vi "THzTimeScan_830_PSD_TA.vi"(0 "input":T1={"Step Number"=0, "Step"=0.0, "Start Position"=0.0, "Time-out"=0, "Lockin Address"="", "Short term \nAverage#"=0, 0, "ESP300 Axis"=0, "Value"="", "Delay"=0.0, "Delay2"=0.0, "savepath"=path "", "Power meter"={"ConexPSD Reference"=refnum, "error out"={"status"=FALSE, "code"=0, "source"=""}, "Component ID"=1}}) -> (1 "loop stop":bool, 2 "x-axis":sgl[](array[numeric]), 3 "y-axis":dbl[](array[numeric]), 4 "ext. out":cluster{dbl[], dbl[], dbl[], dbl[], string[]})   [LabVIEW 2010]
uses:
  C:/Users/NBTP/Desktop/Tai Anh/5. Tools Project/LabVIEW/노트북LabVIEW/THz Time/THz Time(SR830_VC_CONEXAGP_nPt_Shot202_2Pt__LGS/Dll/Newport.CONEXPSD.CommandInterface.DLL
  노트북LabVIEW/THz Time/THz Time(SR830_VC_CONEXAGP_nPt_Shot202_2Pt__LGS/Dll/Newport.CONEXPSD.CommandInterface.DLL
  <vilib>/Utility/file.llb/Write To Spreadsheet File (string).vi
panel:
  out "Total info.":cluster{dbl, dbl, dbl}(graph)
  in  "y offset":dbl
  in  "x offset":dbl
  out "PD pow.":dbl
  out "Y pos.":dbl
  out "X pos.":dbl
  in  "pow. offset":dbl
  out "Pow.":dbl
  out "Array":dbl[](array[numeric])
  out "String":string
  out "Read position":bool
  out "Ask position":bool
  out "Move delay":bool
  out "Read830":bool
  out "Command":string
  out "THz Signal Graph":dbl(graph)
  in  "loop stop":bool
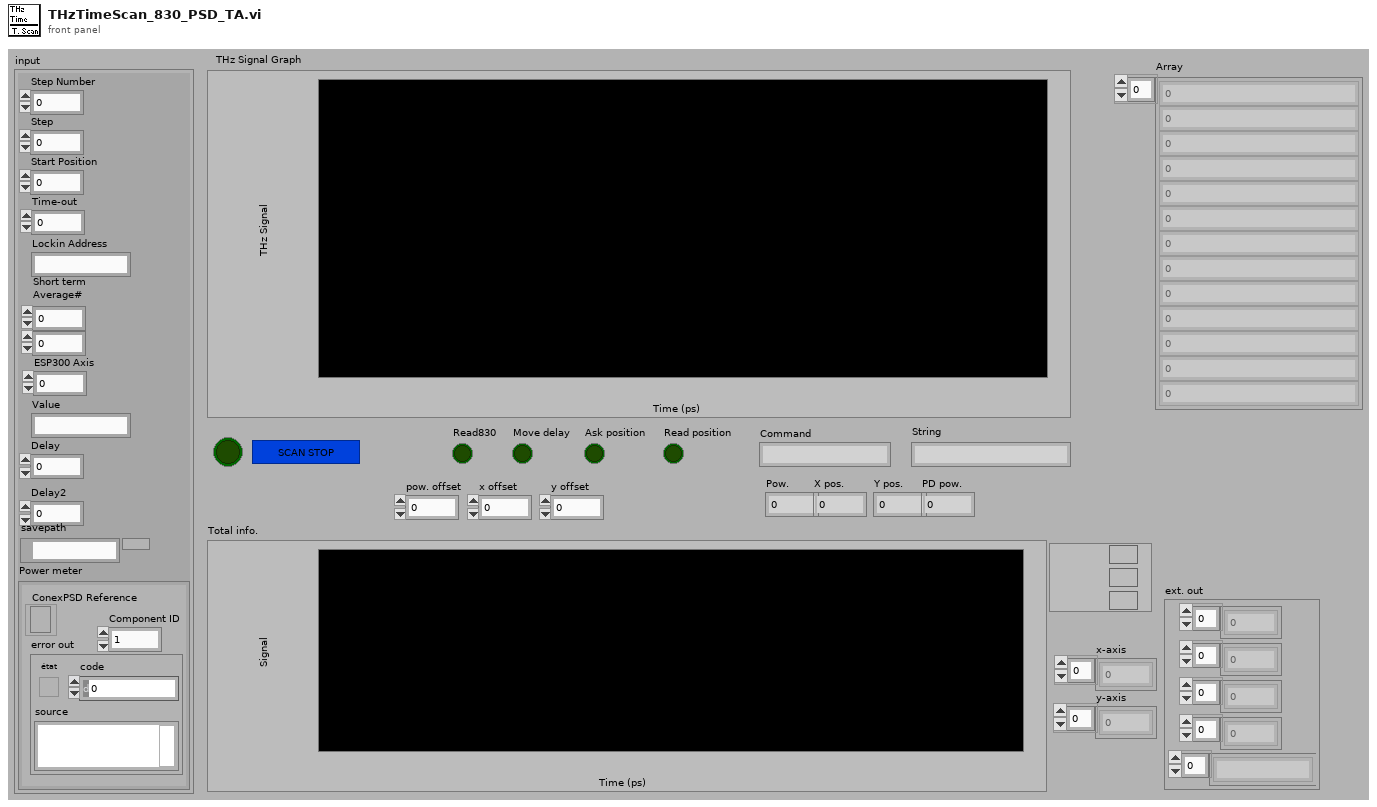
[diagram p1: front panel]
types:
  T1 = cluster{"Step Number":i32, "Step":sgl, "Start Position":sgl, "Time-out":i32, "Lockin Address":string, "Short term \nAverage#":i8, i32, "ESP300 Axis":i8, "Value":string, "Delay":dbl, "Delay2":dbl, "savepath":path, "Power meter":cluster{"ConexPSD Reference":refnum<k24>, "error out":errorcluster, "Component ID":i32}}
  T2 = cluster{"ConexPSD Reference":refnum<k24>, "error out":errorcluster, "Component ID":i32}
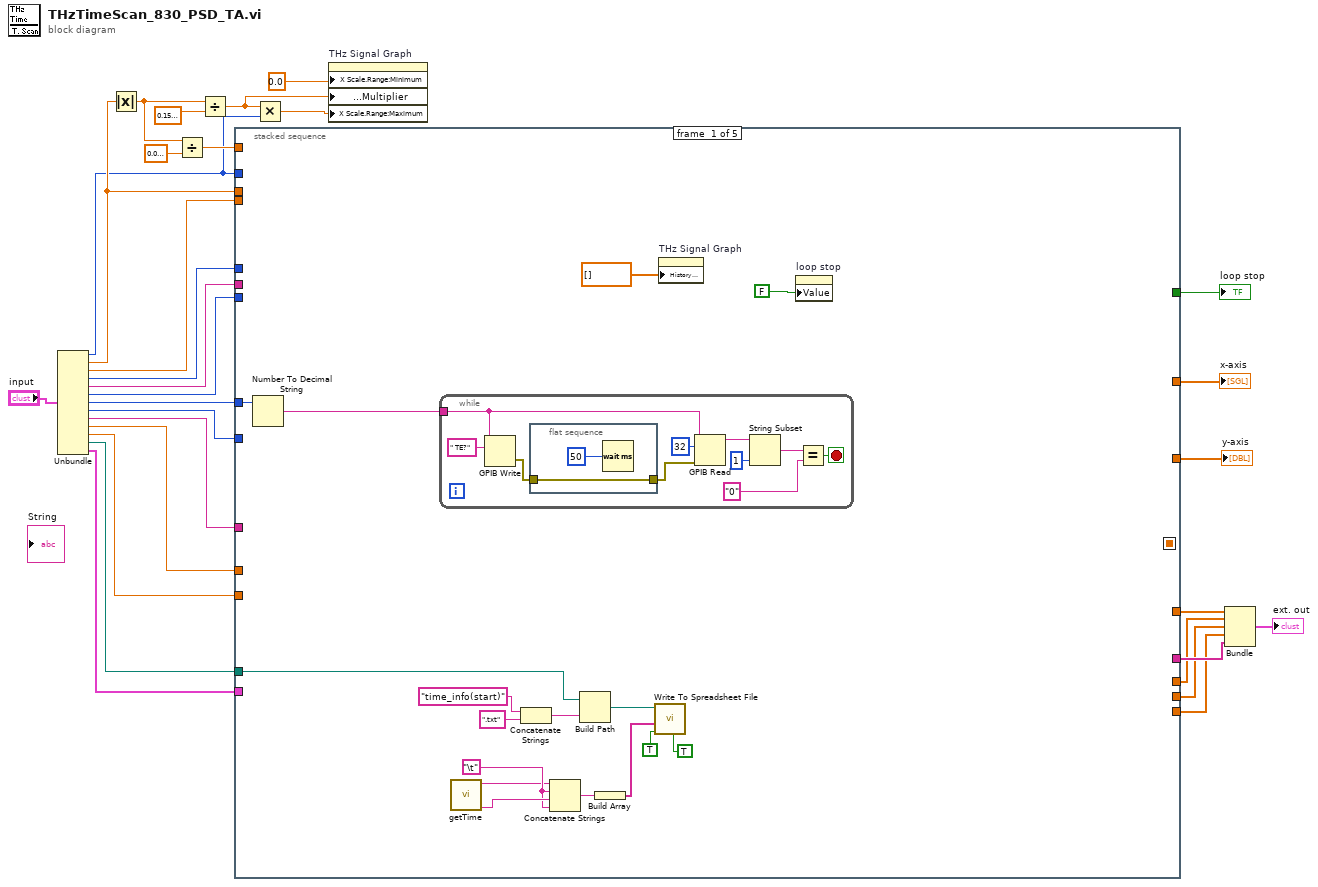
[diagram p0: block diagram]
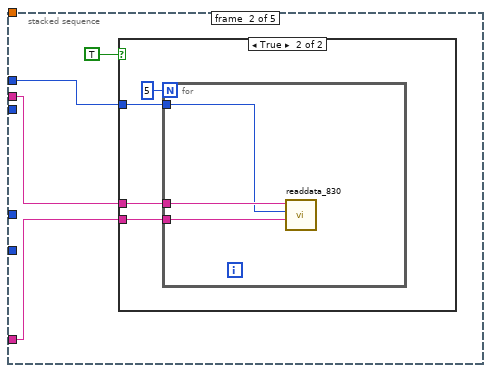
[diagram p2: hidden frame]
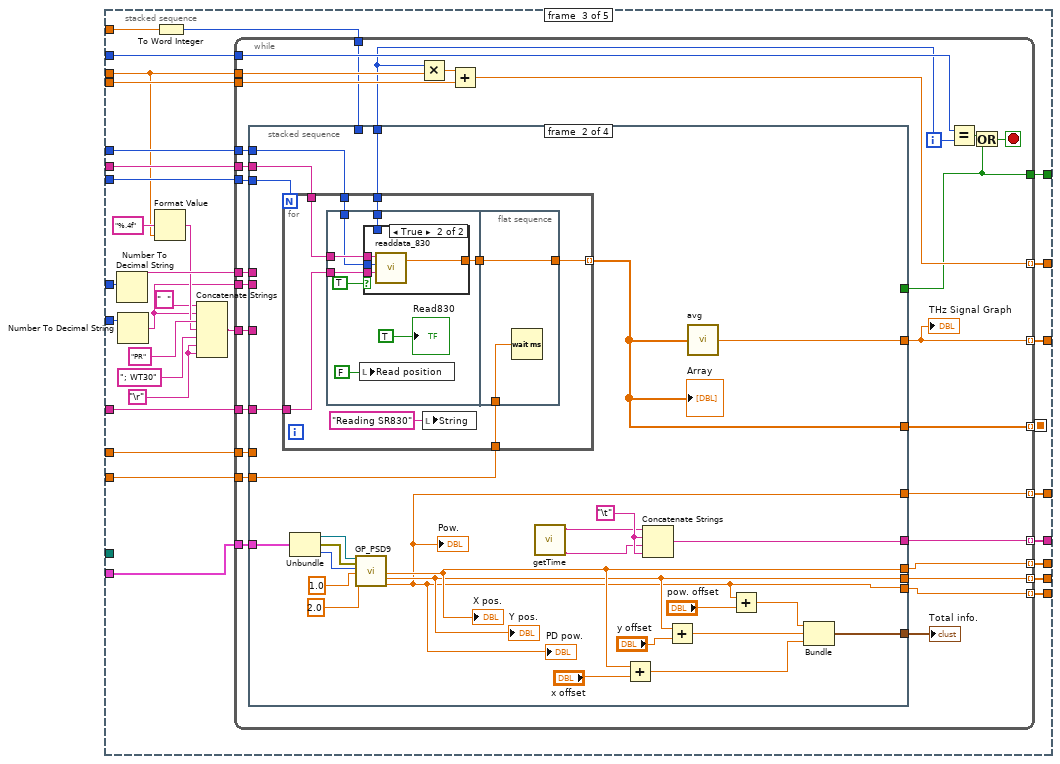
[diagram p4: hidden frame]
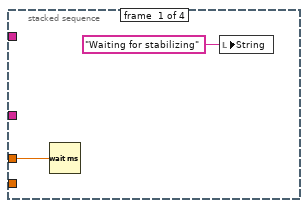
[diagram p5: hidden frame]
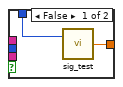
[diagram p6: hidden frame]
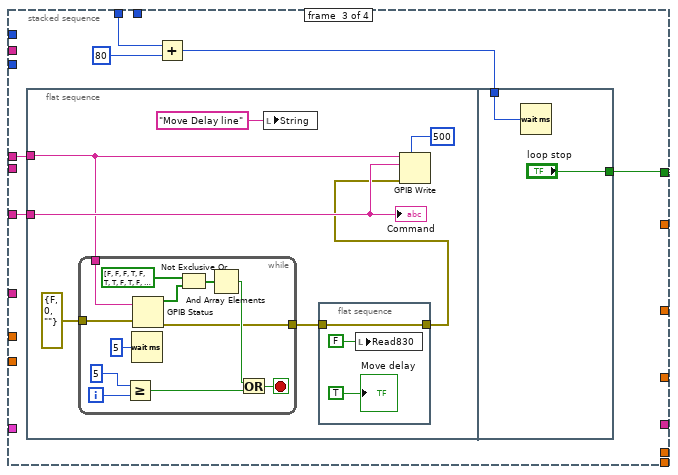
[diagram p7: hidden frame]
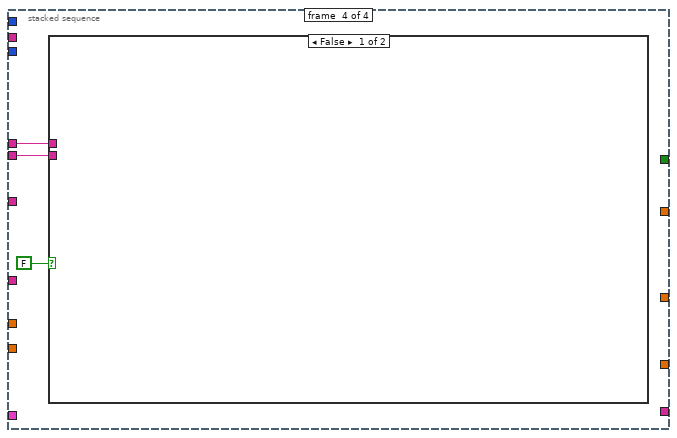
[diagram p8: hidden frame]
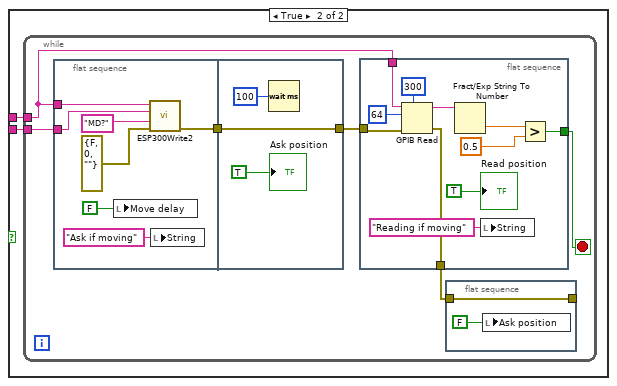
[diagram p9: hidden frame]
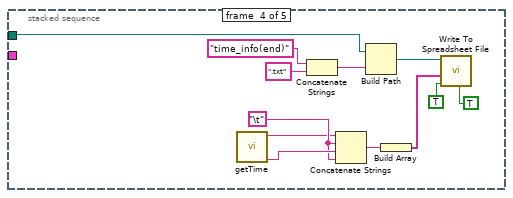
[diagram p10: hidden frame]
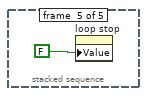
[diagram p11: hidden frame]
diagram:
  n1 = Unbundle("input") -> ("Step Number"=w15:i32, "Step"=w22:sgl, "Start Position"=w21:sgl, "Time-out"=w20:i32, "Lockin Address"=w19:string, "Short term \nAverage#"=w11:i8, w18:i32, "ESP300 Axis"=w17:i8, "Value"=w16:string, "Delay"=w10:dbl, "Delay2"=w9:dbl, "savepath"=w8:path, "Power meter"=w7:T2)
  n2 = Absolute Value(x=w22) -> (abs(x)=w26:sgl)
  n3 = Divide(x=w26, y=sgl 0.004) -> (x/y=w24:sgl)
  n4 = Divide(x=w26, y=sgl 0.15) -> (x/y=w13:sgl)
  n5 = stacked-sequence {
    seq-local: [_ _ w77 _ _] -> [_ _ _ _ _]
    tunnel: w21 -> [_ _ w101 _ _]
    tunnel: w20 -> [_ w62 w100 _ _]
    tunnel: w19 -> [_ w61 w99 _ _]
    tunnel: w11 -> [_ _ w98 _ _]
    tunnel: w18 -> [w44 _ w93 _ _]
    tunnel: w17 -> [_ _ w91 _ _]
    tunnel: w16 -> [_ w60 w83 _ _]
    tunnel: [_ _ w97 _ _] -> w30
    tunnel: [_ _ w96 _ _] -> w29
    tunnel: [_ _ w95 _ _] -> w28
    tunnel: w22 -> [_ _ w89 _ _]
    tunnel: w15 -> [_ _ w94 _ _]
    tunnel: w24 -> [_ _ w88 _ _]
    tunnel: w10 -> [_ _ w79 _ _]
    tunnel: w9 -> [_ _ w78 _ _]
    tunnel: w8 -> [w31 _ _ w248 _]
    tunnel: w7 -> [_ _ w75 _ _]
    tunnel: [_ _ w74 _ _] -> w6
    tunnel: [_ _ w73 _ _] -> w5
    tunnel: [_ _ w72 _ _] -> w4
    tunnel: [_ _ w71 _ _] -> w3
    tunnel: [_ _ w70 _ _] -> w2
    frame #0 {
      w34 = "\t"
      n6 = Number To Decimal String(number=w44) -> (decimal integer string=w43:string)  [unwired: 1 in]
      n7 = while {
        tunnel: w43 -> [w49]
        stop <- w54 stop-if-true
        n8 = GPIB Write(0:w49, 1:" TE?" ("data")) -> (6:w48:errorcluster)  [unwired: 3 in, 1 out]
        n9 = flat-sequence {
          tunnel: w48 -> [w58]
          tunnel: [w58] -> w47
          frame #0 {
            n10 = Wait (ms)(milliseconds to wait=u32 50) -> ()  [unwired: 1 out]
          }
        }
        n11 = GPIB Read(0:w49, 1:32 ("byte count"), 3:w47) -> (5:w53:string)  [unwired: 2 in, 2 out]
        n12 = String Subset(string=w53, length (rest)=1 ("offset (0)")) -> (substring=w51:string)  [unwired: 1 in]
        n13 = Equal?(x=w51, y="0") -> (x = y?=w54:bool)
      }
      n14 = call "getTime.vi"() -> ("시간"=w35:string, "날짜"=w33:string)  [unwired: 10 in]
      n15 = Concatenate Strings("time_info(start)" ("string"), ".txt" ("string")) -> (w41:string)
      n16 = Concatenate Strings(w33, w34, w35, w34) -> (w32:string)
      n17 = Build Path(base path=w31, name or relative path=w41) -> (appended path=w38:path)
      n18 = Build Array(w32) -> (w37:string[])
      n19 = call-poly <vilib>:"Write To Spreadsheet File.vi"("transpose? (no:F)"=TRUE ("transpose?\n(no:F)"), "append to file? (new file:F)"=TRUE ("transpose?\n(no:F)"), "1D data"=w37, "file path (dialog if empty)"=w38) -> ()  [unwired: 4 in, 1 out]
      n20 = property on="THz Signal Graph" class="WFChart (strict)"("History Data"=dbl[] []) -> ()  [unwired: 2 in, 2 out]
      n21 = property on="loop stop" class="Bool (strict)"("Value"=FALSE) -> ()  [unwired: 2 in, 2 out]
    }
    frame #1 {
      n22 = case shown="True" TRUE {
        tunnel: w62 -> [_ w65]
        tunnel: w61 -> [_ w64]
        tunnel: w60 -> [_ w63]
        frame False {
        }
        frame True {
          n23 = for {
            N: 5 -> [_]
            tunnel: w64 -> [w69]
            tunnel: w63 -> [w68]
            tunnel: w65 -> [w67]
            n24 = call "readdata_830.vi"("Command"=w68, "timeout"=w67, "Lockin Address"=w69) -> ()  [unwired: 1 in, 2 out]
          }
        }
      }
    }
    frame #2 {
      w82 = "\r"
      n25 = Number To Decimal String(number=w93) -> (decimal integer string=w92:string)  [unwired: 1 in]
      n26 = Number To Decimal String(number=w91) -> (decimal integer string=w80:string)  [unwired: 1 in]
      n27 = Format Value(format string="%.4f", value (0)=w89) -> (output string=w85:string)  [unwired: 1 in]
      n28 = To Word Integer(number=w88) -> (16bit integer=w87:i16)
      n29 = Concatenate Strings("  " ("string"), w80, "PR" ("Substring"), w85, "; WT30" ("string"), w82, w82) -> (w76:string)
      n30 = while {
        tunnel: [w114] -> w97
        tunnel: [w120] -> w95 mode=indexing
        tunnel: [w126] -> w96 mode=indexing
        tunnel: w94 -> [w125]
        tunnel: w89 -> [w124]
        tunnel: w101 -> [w123]
        tunnel: w100 -> [w115]
        tunnel: w99 -> [w122]
        tunnel: w98 -> [w121]
        tunnel: w92 -> [w119]
        tunnel: w76 -> [w118]
        tunnel: w87 -> [w117]
        tunnel: w83 -> [w116]
        tunnel: w80 -> [w113]
        tunnel: w79 -> [w112]
        tunnel: w78 -> [w111]
        tunnel: [w110] -> w77 mode=indexing
        tunnel: w75 -> [w108]
        tunnel: [w107] -> w71 mode=indexing
        tunnel: [w106] -> w72 mode=indexing
        tunnel: [w105] -> w70 mode=indexing
        tunnel: [w103] -> w74 mode=indexing
        tunnel: [w102] -> w73 mode=indexing
        i -> [w109]
        stop <- w129 stop-if-true
        n31 = stacked-sequence {
          tunnel: w122 -> [_ w156 _ _]
          tunnel: [_ w158 _ _] -> w120
          tunnel: w121 -> [_ w159 _ _]
          tunnel: w119 -> [_ _ w188 w216]
          tunnel: w118 -> [_ _ w189 _]
          tunnel: w117 -> [_ _ w187 _]
          tunnel: w116 -> [_ w157 _ _]
          tunnel: w115 -> [_ w155 _ _]
          tunnel: [_ _ w184 _] -> w114
          tunnel: w113 -> [_ _ _ w215]
          tunnel: w112 -> [w131 _ _ _]
          tunnel: w111 -> [_ w154 _ _]
          tunnel: [_ w153 _ _] -> w110
          tunnel: w109 -> [_ w152 _ _]
          tunnel: w108 -> [_ w139 _ _]
          tunnel: [_ w135 _ _] -> w103
          tunnel: [_ w138 _ _] -> w102
          tunnel: [_ w137 _ _] -> w106
          tunnel: [_ w136 _ _] -> w107
          tunnel: [_ w135 _ _] -> w105
          tunnel: [_ w134 _ _] -> w104
          frame #0 {
            n32 = Wait (ms)(milliseconds to wait=w131) -> ()  [unwired: 1 out]
            n33 = local write "String"("Waiting for stabilizing" ("String")) -> ()
          }
          frame #1 {
            w146 = "\t"
            n34 = for {
              N: w159 -> [_]
              tunnel: w156 -> [w164]
              tunnel: w155 -> [w167]
              tunnel: [w166] -> w153 mode=indexing
              tunnel: w157 -> [w165]
              tunnel: w154 -> [w161]
              tunnel: w152 -> [w160]
              n35 = flat-sequence {
                tunnel: w167 -> [w171]
                tunnel: w165 -> [w172]
                tunnel: w164 -> [w173]
                tunnel: [w170] -> w162
                tunnel: w160 -> [w168]
                tunnel: [w183] -> w166
                tunnel: w162 -> [w183]
                tunnel: w161 -> [w182]
                frame #0 {
                  n36 = local write "Read position"(FALSE ("Read position")) -> ()
                  n37 = case shown="True" TRUE {
                    tunnel: w173 -> [_ w181]
                    tunnel: w172 -> [_ w180]
                    tunnel: w171 -> [_ w179]
                    tunnel: [w177 w178] -> w170
                    tunnel: w168 -> [w176 _]
                    frame False {
                      n38 = call "sig_test.vi"("index (row)"=w176) -> ("element"=w177:dbl)  [unwired: 1 in]
                    }
                    frame True {
                      n39 = call "readdata_830.vi"("Command"=w180, "timeout"=w179, "Lockin Address"=w181) -> ("Data"=w178:dbl)  [unwired: 1 in, 1 out]
                    }
                  }
                  "Read830" <- TRUE ("Read830")
                }
                frame #1 {
                  n40 = Wait (ms)(milliseconds to wait=w182) -> ()  [unwired: 1 out]
                }
              }
              n41 = local write "String"("Reading SR830" ("String")) -> ()
            }
            "Array" <- w153
            n42 = Unbundle(w139) -> ("ConexPSD Reference"=w151:refnum<k24>, "error out"=w150:errorcluster, "Component ID"=w149:i32)
            n43 = call "GP_PSD9.vi"("ConexPSD Reference"=w151, "error out"=w150, "Component ID"=w149, "Adress"=1.0, "shot average"=2.0) -> ("PositionX"=w137:dbl, "PositionY"=w136:dbl, "LaserPower"=w135:dbl)  [unwired: 8 in, 4 out]
            "Pow." <- w135
            "X pos." <- w137
            "Y pos." <- w136
            "PD pow." <- w135
            n44 = call "getTime.vi"() -> ("시간"=w132:string, "날짜"=w133:string)  [unwired: 10 in]
            n45 = Add(x=w137, y="x offset") -> (x+y=w143:dbl)
            n46 = Concatenate Strings(w133, w146, w132, w146) -> (w138:string)
            n47 = Add(x=w136, y="y offset") -> (x+y=w144:dbl)
            n48 = call "avg.vi"("Array"=w153) -> ("Numeric"=w158:dbl)
            n49 = Add(x=w135, y="pow. offset") -> (x+y=w145:dbl)
            n50 = Bundle(w145, w144, w143) -> (w134:cluster{dbl, dbl, dbl})  [unwired: 1 in]
          }
          frame #2 {
            n51 = flat-sequence {
              tunnel: w189 -> [w196]
              tunnel: w188 -> [w194]
              tunnel: w186 -> [w212]
              tunnel: ["loop stop"] -> w184
              frame #0 {
                n52 = while {
                  tunnel: errorcluster {"status"=FALSE, "code"=0, "source"=""} ("error in (no error)") -> [w211]
                  tunnel: [w201] -> w191
                  tunnel: w194 -> [w200]
                  i -> [w210]
                  stop <- w207 stop-if-true
                  n53 = Greater Or Equal?(x=5, y=w210) -> (x >= y?=w208:bool)
                  n54 = Wait (ms)(milliseconds to wait=u32 5) -> ()  [unwired: 1 out]
                  n55 = GPIB Status(0:w200, 1:w211) -> (2:w205:bool[], 5:w201:errorcluster)  [unwired: 2 out]
                  n56 = Not Exclusive Or(1:w205, 2:bool[] [FALSE, FALSE, FALSE, TRUE, FALSE, TRUE, TRUE, FALSE, TRUE, FALSE, FALSE, FALSE, FALSE, FALSE, FALSE, FALSE] ("status 2")) -> (0:w204:bool[])
                  n57 = And Array Elements(Boolean array=w204) -> (logical AND=w203:bool)
                  n58 = Or(x=w203, y=w208) -> (x .or. y?=w207:bool)
                }
                n59 = local write "String"("Move Delay line" ("String")) -> ()
                n60 = flat-sequence {
                  tunnel: [w199] -> w192
                  tunnel: w191 -> [w199]
                  frame #0 {
                    n61 = local write "Read830"(FALSE ("Read830")) -> ()
                    "Move delay" <- TRUE ("Move delay")
                  }
                }
                n62 = GPIB Write(0:w194, 1:w196, 3:w192, 4:500 ("timeout ms (488.2 global)")) -> ()  [unwired: 1 in, 2 out]
                "Command" <- w196
              }
              frame #1 {
                n63 = Wait (ms)(milliseconds to wait=w212) -> ()  [unwired: 1 out]
              }
            }
            n64 = Add(x=w187, y=i16 80) -> (x+y=w186:i16)
          }
          frame #3 {
            n65 = case shown="False" FALSE {
              tunnel: w216 -> [_ w218]
              tunnel: w215 -> [_ w217]
              frame False {
              }
              frame True {
                n66 = while {
                  tunnel: w218 -> [w220]
                  tunnel: w217 -> [w224]
                  stop <- w222 stop-if-true
                  n67 = flat-sequence {
                    tunnel: w224 -> [w238]
                    tunnel: w220 -> [w241]
                    tunnel: [w242] -> w221
                    tunnel: [w247] -> w223
                    tunnel: w221 -> [w247]
                    frame #0 {
                      n68 = local write "Move delay"(FALSE ("Move delay")) -> ()
                      n69 = call "ESP300Write2.vi"("error in (no error)"=errorcluster {"status"=FALSE, "code"=0, "source"=""}, "Command"="MD?", "ESP300 Channel"=w238, "ESP300 Address"=w241) -> ("error out"=w242:errorcluster)  [unwired: 3 in]
                      n70 = local write "String"("Ask if moving" ("String")) -> ()
                    }
                    frame #1 {
                      n71 = Wait (ms)(milliseconds to wait=u32 100) -> ()  [unwired: 1 out]
                      "Ask position" <- TRUE ("Ask position")
                    }
                  }
                  n72 = flat-sequence {
                    tunnel: w223 -> [w237]
                    tunnel: [w234] -> w222
                    tunnel: w220 -> [w230]
                    tunnel: [w228] -> w219
                    frame #0 {
                      n73 = GPIB Read(0:w230, 1:64 ("byte count"), 3:w237, 4:300 ("timeout ms (488.2 global)")) -> (5:w233:string, 7:w228:errorcluster)  [unwired: 1 in, 1 out]
                      n74 = Fract/Exp String To Number(string=w233) -> (number=w232:dbl)  [unwired: 3 in, 1 out]
                      n75 = local write "String"("Reading if moving" ("String")) -> ()
                      n76 = Greater?(x=w232, y=0.5) -> (0:w234:bool)
                      "Read position" <- TRUE ("Read position")
                    }
                  }
                  n77 = flat-sequence {
                    tunnel: [w226] -> _
                    tunnel: w219 -> [w226]
                    frame #0 {
                      n78 = local write "Ask position"(FALSE ("Ask position")) -> ()
                    }
                  }
                }
              }
            }
          }
        }
        "THz Signal Graph" <- w120
        "Total info." <- w104
        n79 = Multiply(x=w109, y=w124) -> (x*y=w127:sgl)
        n80 = Add(x=w127, y=w123) -> (x+y=w126:sgl)
        n81 = Equal?(x=w125, y=w109) -> (x = y?=w128:bool)
        n82 = Or(x=w128, y=w114) -> (x .or. y?=w129:bool)
      }
    }
    frame #3 {
      w251 = "\t"
      n83 = call "getTime.vi"() -> ("시간"=w252:string, "날짜"=w250:string)  [unwired: 10 in]
      n84 = Concatenate Strings("time_info(end)" ("string"), ".txt" ("string")) -> (w258:string)
      n85 = Concatenate Strings(w250, w251, w252, w251) -> (w249:string)
      n86 = Build Path(base path=w248, name or relative path=w258) -> (appended path=w255:path)
      n87 = Build Array(w249) -> (w254:string[])
      n88 = call-poly <vilib>:"Write To Spreadsheet File.vi"("transpose? (no:F)"=TRUE ("transpose?\n(no:F)"), "append to file? (new file:F)"=TRUE ("transpose?\n(no:F)"), "1D data"=w254, "file path (dialog if empty)"=w255) -> ()  [unwired: 4 in, 1 out]
    }
    frame #4 {
      n89 = property on="loop stop" class="Bool (strict)"("Value"=FALSE) -> ()  [unwired: 2 in, 2 out]
    }
  }
  "loop stop" <- w30
  "x-axis" <- w29
  "y-axis" <- w28
  n90 = Multiply(x=w13, y=w15) -> (x*y=w12:sgl)
  n91 = property on="THz Signal Graph" class="WFChart (strict)"("X Scale.Range:Minimum"=0.0, "X Scale.Offset and Multiplier:Multiplier"=w13, "X Scale.Range:Maximum"=w12) -> ()  [unwired: 2 in, 2 out]
  n92 = Bundle(w6, w4, w3, w2, w5) -> (→"ext. out":cluster{dbl[], dbl[], dbl[], dbl[], string[]})  [unwired: 1 in]
